vi "SRS8XX_auto_read2.vi"() -> ()   [LabVIEW 2020]
panel:
  in  "SR 8XX settings":T1(array[cluster])=[{"Instrument Address"="GPIB0::1::INSTR", "parameters"=[0.9, 0.1, 1e-07, 1e-05, 0.0], "channel"=enum."X channel only", "enable"=TRUE, "lockin"=enum."SRS 830"}, {"Instrument Address"="GPIB0::2::INSTR", "parameters"=[0.9, 0.1, 1e-07, 1e-05, 0.0], "channel"=enum."X channel only", "enable"=TRUE, "lockin"=enum."SRS 830"}, {"Instrument Address"="GPIB0::3::INSTR", "parameters"=[0.9, 0.1, 1e-07, 1e-05, 0.0], "channel"=enum."X channel only", "enable"=TRUE, "lockin"=enum."SRS 830"}, {"Instrument Address"="GPIB0::4::INSTR", "parameters"=[0.9, 0.1, 1e-07, 1e-05, 0.0], "channel"=enum."X channel only", "enable"=TRUE, "lockin"=enum."SRS 830"}] {"parameters" format="%.2e"}
  out "elapsed time (ms)":u32
  in  "stop":bool
  in  "clear devices\non errors":bool
  out "VISA error?":bool
  out "CH1 and Ch2 output":cluster{"Array":dbl[], "Boolean":bool}[](array[cluster]) {"Array" format="%#_3e"}
  out "Data":dbl[](array[numeric])=[-0.00093841552734, -0.00033187866211, -1.9930615736e-07, -1.0389822336e-09, -0.00070953369141, -0.00042343139648]
  in  "read data?":enum16{"None", "X only", "X Y"}(ring)
  in  "interval between \nreading/sensitivity adjustment (msec)":i32
  # "(works better with read XY data\noption ON)"
  # "Error"
  # "1. Connect CH1 OUT to AUX1 IN\n2. Connect CH2 OUT to AUX2 IN\n3. Set CH1 OUTPUT to X\n4. Set CH2 OUTPUT to Y\n\nThis VI reads the AO of the X and Y channels (10 V for full scale)\nand adjust sensitivity to have the desired sensitivity\n\nparameter 0\n  : upper limit for lowering sensitivity\n  ex) 0.9 -> decrease sensitivy when signal\n      reached 90% of the sensitivity\nparameter 1\n   : lower limit for increasing sensitivity\nparameter 2\n     : highest sensitivity\n     sensitivity will not be higher than this value"
  # "highest\nsensitivity(V)"
  # "upper\nlimit"
  # "lower\nlimit"
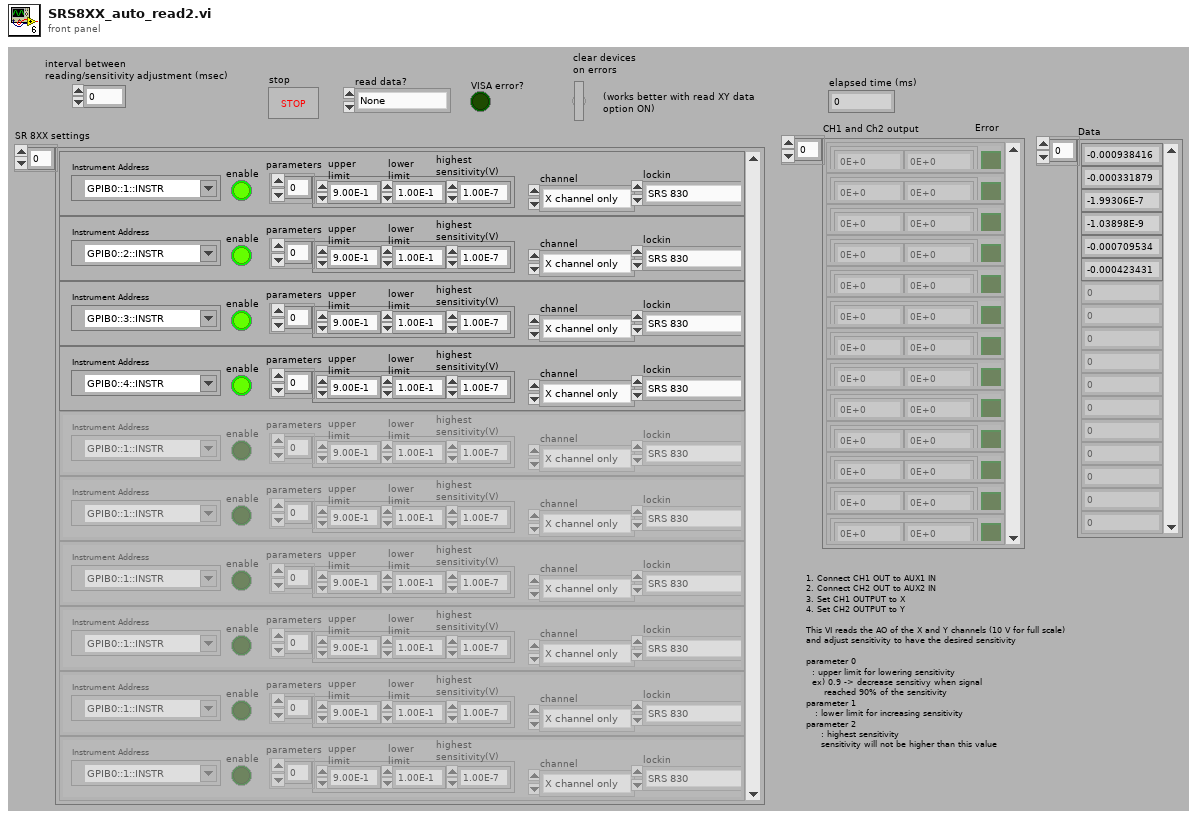
[diagram p1: front panel]
types:
  T1 = cluster{"Instrument Address":refnum<visa-resource-name>, "parameters":dbl[], "channel":enum16{"R ", "X channel only", "Y channel only"}, "enable":bool, "lockin":enum16{"SRS 830", "SRS 86X", "SigRec 72XX"}}[]
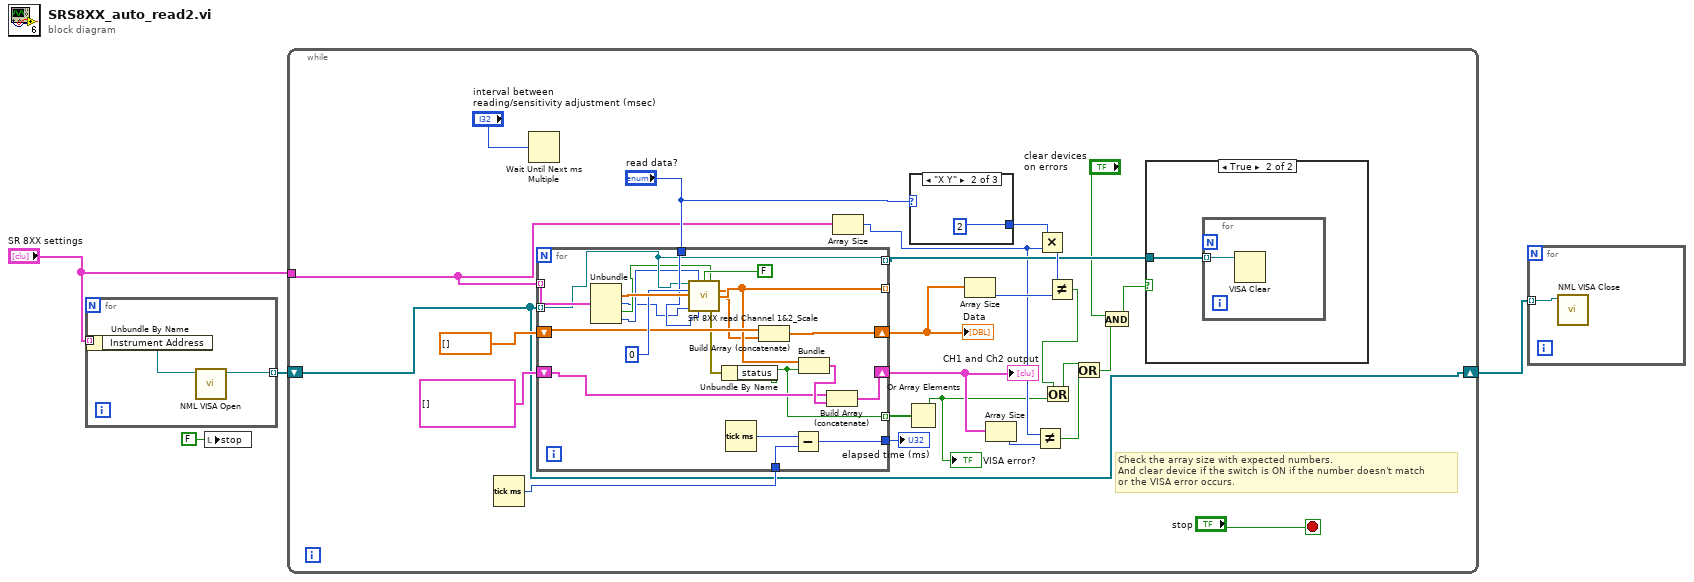
[diagram p0: block diagram]
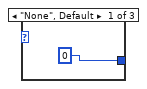
[diagram p3: hidden frame]
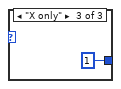
[diagram p4: hidden frame]
diagram:
  n1 = for {
    tunnel: "SR 8XX settings" -> [w7] mode=indexing
    tunnel: [w5] -> w3 mode=indexing
    n2 = Unbundle By Name(w7) -> ("Instrument Address"=w6:refnum<visa-resource-name>)
    n3 = call "NML VISA Open.vi"("VISA resource name"=w6) -> ("VISA resource name out"=w5:refnum<visa-resource-name>)  [unwired: 9 in, 1 out]
  }
  n4 = local write "stop"(FALSE ("stop")) -> ()
  n5 = while {
    tunnel: "SR 8XX settings" -> [w9]
    shift-right: [w8] -> w2
    shift-left: w3 -> [w8]
    stop <- "stop" stop-if-true
    # "Check the array size with expected numbers.\nAnd clear device if the switch is ON if the number doesn't match\nor the VISA error occurs."
    n6 = Tick Count (ms)() -> (millisecond timer value=w11:u32)
    n7 = Wait Until Next ms Multiple(millisecond multiple="interval between \nreading/sensitivity adjustment (msec)") -> ()  [unwired: 1 out]
    n8 = for {
      tunnel: w9 -> [w54] mode=indexing
      tunnel: [w53] -> _ mode=indexing
      shift-right: [w56] -> w25
      shift-left: dbl[] [] -> [w55]
      shift-right: [w50] -> w19
      shift-left: cluster{"CH Output":dbl[], bool}[] [] -> [w49]
      tunnel: [w47] -> w29 mode=indexing
      tunnel: "read data?" -> [w46]
      tunnel: [w42] -> w23 mode=indexing
      tunnel: w11 -> [w44]
      tunnel: [w43] -> w10
      tunnel: w8 -> [w42] mode=indexing
      n9 = Unbundle(w54) -> ("parameters"=w58:dbl[], "channel"=w38:enum16{"R ", "X channel only", "Y channel only"}, "enable"=w39:bool, "lockin"=w40:enum16{"SRS 830", "SRS 86X", "SigRec 72XX"})  [unwired: 1 out]
      n10 = call "SR 8XX read Channel 1&2_Scale.vi"("Instrument Address"=w42, "lockin"=w40, "close VISA ref."=FALSE ("close VI"), "enable auto?"=w39, "Point #"=0, "parameters_x"=w58, "channel"=w38, "read data"=w46) -> ("Data"=w52:dbl[], "CH Output"=w53:dbl[], "error in (no error) 2"=w48:errorcluster)  [unwired: 2 in, 3 out]
      n11 = Unbundle By Name(w48) -> ("status"=w47:bool)
      n12 = Tick Count (ms)() -> (millisecond timer value=w45:u32)
      n13 = Build Array (concatenate)(w55, w52) -> (w56:dbl[])
      n14 = Subtract(x=w45, y=w44) -> (x-y=w43:u32)
      n15 = Bundle("CH Output"=w53, "status"=w47) -> (w51:cluster{"CH Output":dbl[], "status":bool})  [unwired: 1 in]
      n16 = Build Array (concatenate)(w49, w51) -> (w50:cluster{"CH Output":dbl[], "status":bool}[])
    }
    "Data" <- w25
    "CH1 and Ch2 output" <- w19
    "elapsed time (ms)" <- w10
    n17 = Array Size(array=w9) -> (size(s)=w17:i32)
    n18 = Or Array Elements(Boolean array=w29) -> (logical OR=w15:bool)
    "VISA error?" <- w15
    n19 = case shown="\"X Y\"" "read data?" {
      tunnel: [0 2 1] -> w28
      frame "None", Default {
      }
      frame "X Y" {
      }
      frame "X only" {
      }
    }
    n20 = Array Size(array=w25) -> (size(s)=w27:i32)
    n21 = Array Size(array=w19) -> (size(s)=w18:i32)
    n22 = Not Equal?(x=w17, y=w18) -> (x != y?=w16:bool)
    n23 = Multiply(x=w28, y=w17) -> (x*y=w26:i32)
    n24 = Not Equal?(x=w26, y=w27) -> (x != y?=w21:bool)
    n25 = Or(x=w21, y=w15) -> (x .or. y?=w14:bool)
    n26 = Or(x=w14, y=w16) -> (x .or. y?=w13:bool)
    n27 = And(x="clear devices\non errors", y=w13) -> (x .and. y?=w20:bool)
    n28 = case shown="True" w20 {
      tunnel: w23 -> [_ w33]
      frame False {
      }
      frame True {
        n29 = for {
          tunnel: w33 -> [w34] mode=indexing
          n30 = VISA Clear(VISA resource name=w34) -> ()  [unwired: 1 in, 2 out]
        }
      }
    }
  }
  n31 = for {
    tunnel: w2 -> [w59] mode=indexing
    n32 = call "NML VISA Close.vi"("VISA resource name"=w59) -> ()  [unwired: 10 in, 1 out]
  }
